vi "Read_Wav.vi"(8 "error in (no error)":errorcluster, 11 "Path to wav":path) -> (0 "error out":errorcluster, 3 "wf":waveform(dbl)(graph))   [LabVIEW 2020]
uses:
  Controls/Wave2STFT_Cfg.ctl
  <vilib>/addons/_XControls/Colormap/SVX Colormap.xctl
  <vilib>/sound2/lvsound2.llb/Sound File Position.ctl
  <vilib>/sound2/lvsound2.llb/Sound File Read Open.vi
  <vilib>/sound2/lvsound2.llb/Sound File Read (DBL).vi
panel:
  out "Spectrogram":T1(xcontrol)={"spectral map"=array79x512[40448 elements], "X scale"={"offset"=0.0, "multiplier"=0.0128}, "Y scale"={"offset"=0.0, "multiplier"=15.625}, "attribute"=variant("NI_OAT_Plot_Type"=variant(enum16{"Frequency-Time", "Time-Frequency", "Order-Time", "Time-Order", "Frequency-RPM", "RPM-Frequency", "Order-RPM", "RPM-Order"} enum."Frequency-Time"))} caption="Colormap"
  in  "STFT Config":T2={"FFT block size"=1024, "window"=3, "time segment"={"from [s]"=-1.0, "to [s]"=-1.0, "time increment"=20.0, "time increment units (%)"=enum."%"}, "dB On (T)"=TRUE, "Dynamic Range(dB)"=80.0, "Mel?"=TRUE} {"window" items=["None "=0, "Hanning"=1, "Hamming"=2, "Blackman-Harris"=3, "Exact Blackman"=4, "Blackman"=5, "Flat Top"=6, "4 Term B-Harris "=7, "7 Term B-Harris"=8, "Low Sidelobe"=9, "Blackman Nuttall"=11]}
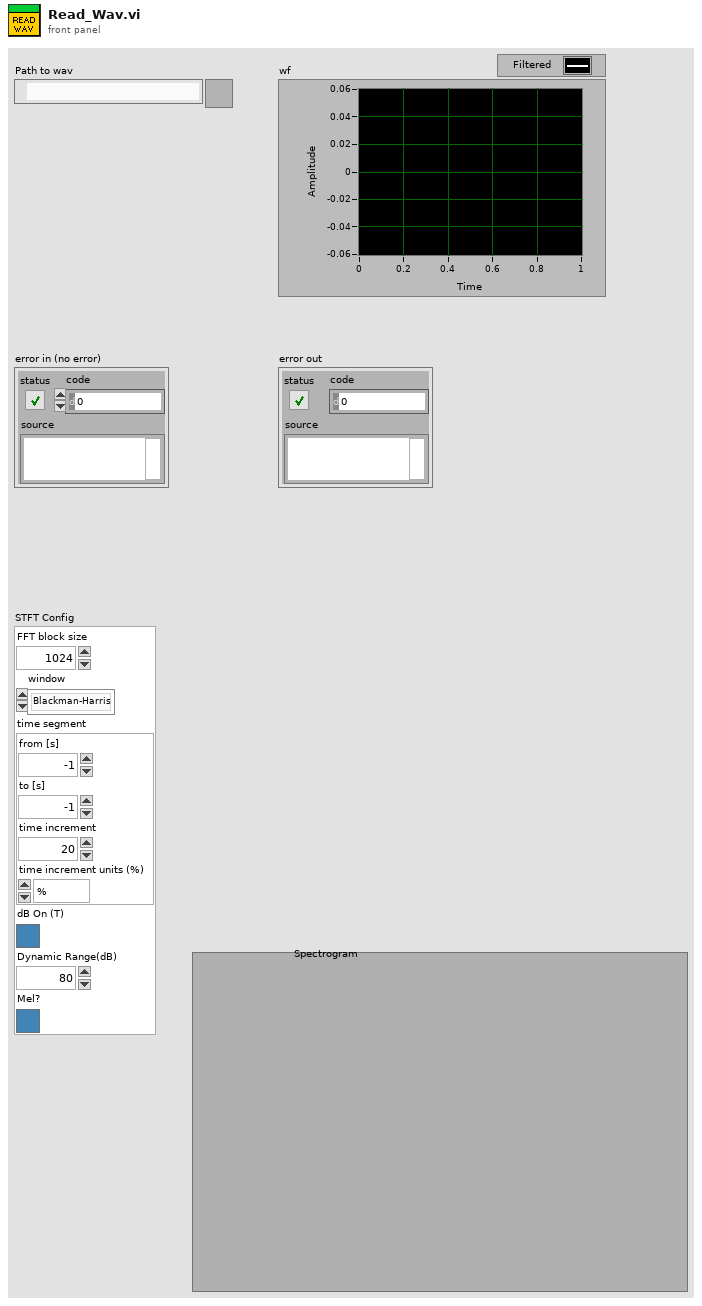
[diagram p1: front panel]
types:
  T1 = cluster{"spectral map":dbl[][], "X scale":cluster{"offset":dbl, "multiplier":dbl}, "Y scale":cluster{"offset":dbl, "multiplier":dbl}, "attribute":variant}
  T2 = typedef "Wave2STFT_Cfg.ctl" = cluster{"FFT block size":i32, "window":u16, "time segment":cluster{"from [s]":dbl, "to [s]":dbl, "time increment":dbl, "time increment units (%)":enum16{"%", "s", "ms"}}, "dB On (T)":bool, "Dynamic Range(dB)":sgl, "Mel?":bool}
  T3 = typedef "Sound File Position.ctl" = u16
  T4 = typedef "Sound File Refnum.ctl" = refnum<file>
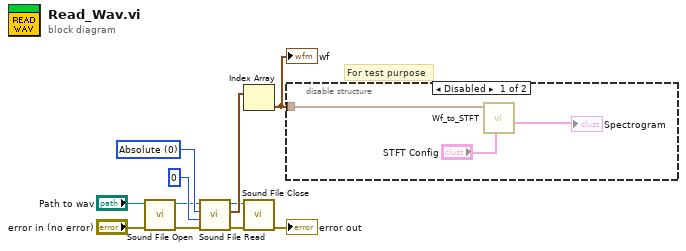
[diagram p0: block diagram]
diagram:
  w8 = T3 0 items=["Absolute"=0, "Relative"=2] ("position mode")
  # "For test purpose"
  n1 = call-poly <vilib>:"Sound File Open.vi"("error in (no error)"="error in (no error)", "path"="Path to wav") -> ("error out"=w5:errorcluster, "sound file refnum"=w6:T4)  [unwired: 8 in]
  n2 = call-poly <vilib>:"Sound File Read.vi"("error in (no error)"=w5, "position offset"=0, "position mode"=w8, "sound file refnum"=w6) -> ("error out"=w9:errorcluster, "data"=w11:waveform(dbl)[], "sound file refnum out"=w10:T4)  [unwired: 3 in, 2 out]
  n3 = Index Array(array=w11) -> (element=w1:waveform(dbl))  [unwired: 1 in]
  "wf" <- w1
  n4 = call <vilib>:"Sound File Close.vi"("error in (no error)"=w9, "sound file refnum"=w10) -> ("error out"=→"error out":errorcluster)  [unwired: 9 in]
  n5 = disable-structure shown="Disabled" {
    disable-tunnel: w1 -> [w14 _]
    frame Disabled {
      n6 = call "Wf_to_STFT.vi"("STFT Config"="STFT Config", "WF"=w14) -> ("STFT"=→"Spectrogram":T1)  [unwired: 7 in, 2 out]
    }
    frame Enabled {
    }
  }
